vi "monochromatorCommandToggleShutter.vi"(8 "error in":errorcluster, 11 "monochromator":refnum<k24>) -> (0 "error out":errorcluster, 2 "shutterAfterToggle":bool, 3 "monochromator":refnum<k24>)   [LabVIEW 2009]
doc: "Check status of the shutter and flip it"
uses:
  C:/Users/anderson.chen/Desktop/Software Development/Cornerstone Series API (LV9)/Cornerstone DLL/Cornerstone.dll
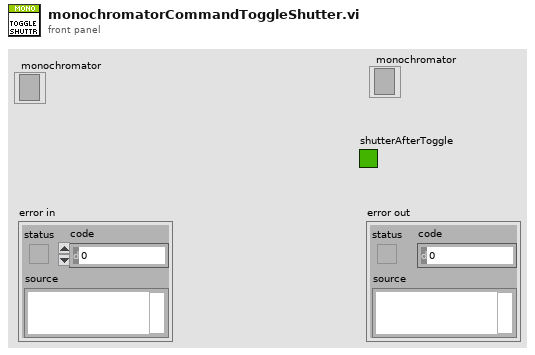
[diagram p1: front panel]
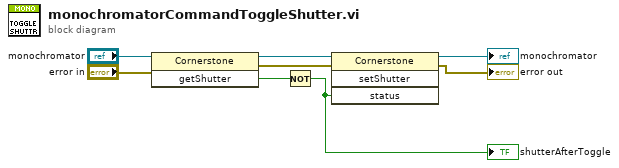
[diagram p0: block diagram]
diagram:
  n1 = invoke class="Cornerstone" method="getShutter"(reference="monochromator", error in="error in") -> (reference out=w7:refnum<k24>, error out=w4:errorcluster, "getShutter"=w2:bool)  [unwired: 1 in]
  n2 = Not(x=w2) -> (.not. x?=w1:bool)
  "shutterAfterToggle" <- w1
  n3 = invoke class="Cornerstone" method="setShutter"(reference=w7, error in=w4, "status"=w1) -> (reference out=→"monochromator":refnum<k24>, error out=→"error out":errorcluster)  [unwired: 1 in, 2 out]
